vi "Clear.vi"(8 "error in (no error)":errorcluster caption="错误输入（无错误）", 11 "ArrayListClass 输入":refnum<class "ArrayListClass.lvclass"> caption="DNL_LabVIEW Object in") -> (0 "error out":errorcluster caption="错误输出", 3 "ArrayListClass 输出":refnum<class "ArrayListClass.lvclass"> caption="DNL_LabVIEW Object out")   [LabVIEW 2012, in "ArrayListClass.lvclass"]
uses:
  ArrayListClass.lvclass
  ArrayListClass.lvclass/ArrayListClass.ctl
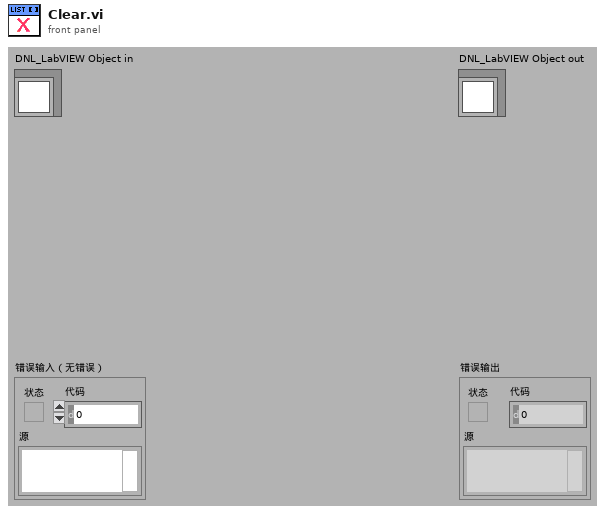
[diagram p1: front panel]
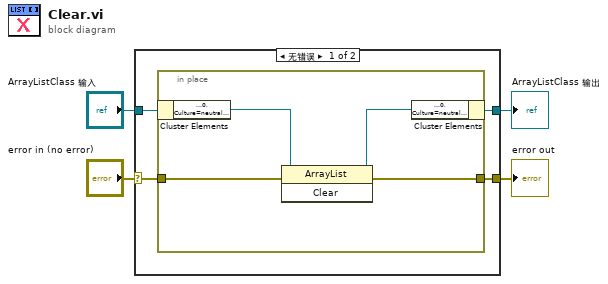
[diagram p0: block diagram]
diagram:
  n1 = case shown="无错误" "error in (no error)" {
    selector: "error in (no error)" -> [w8 w14]
    tunnel: [w7 w14] -> w3
    tunnel: [w5 w13] -> w1
    tunnel: "ArrayListClass 输入" -> [w6 w13]
    frame No Error {
      n2 = in-place {
        in-place-border: w8 -> [w11]
        in-place-border: [w10] -> w7
        n3 = in-place-cluster #1(w6) -> ("ArrayList"=w9:refnum<k24>)
        n4 = invoke class="ArrayList" method="Clear"(reference=w9, error in=w11) -> (reference out=w12:refnum<k24>, error out=w10:errorcluster)  [unwired: 1 in, 1 out]
        n5 = in-place-cluster #1("ArrayList"=w12) -> (w5:refnum<class "ArrayListClass.lvclass">)
      }
    }
    frame Error {
    }
  }
  "error out" <- w3
  "ArrayListClass 输出" <- w1
